vi "ManipulaEventos.vi"(10 "Error en fechas?":bool, 11 "Data In":string[][](array[string])) -> ()   [LabVIEW 2018]
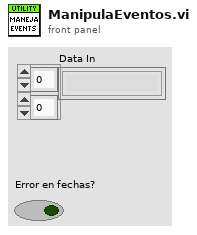
[diagram p1: front panel]
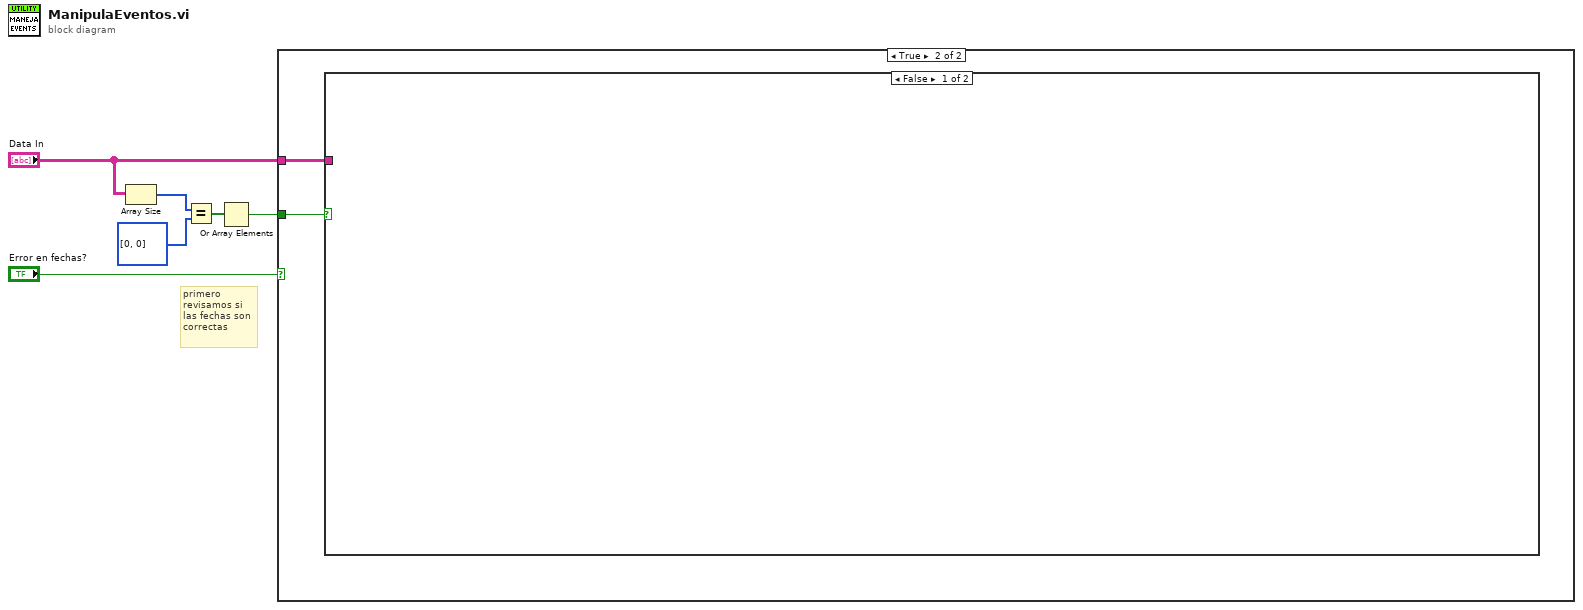
[diagram p0: block diagram]
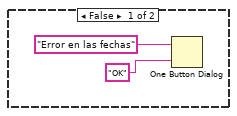
[diagram p2: hidden frame]
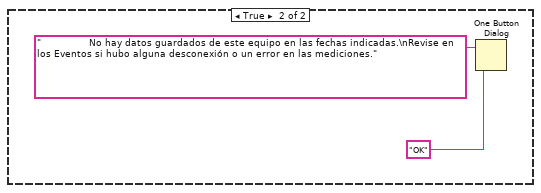
[diagram p3: hidden frame]
diagram:
  # "primero \nrevisamos si \nlas fechas son\ncorrectas"
  n1 = Array Size(array="Data In") -> (size(s)=w6:i32[])
  n2 = Equal?(x=w6, y=i32[] [0, 0] ("size(s)")) -> (x = y?=w4:bool[])
  n3 = Or Array Elements(Boolean array=w4) -> (logical OR=w3:bool)
  n4 = case shown="True" "Error en fechas?" {
    tunnel: w3 -> [_ w10]
    tunnel: "Data In" -> [_ w9]
    frame False {
      n5 = One Button Dialog(message="Error en las fechas", button name ("OK")="OK") -> ()  [unwired: 1 out]
    }
    frame True {
      n6 = case shown="False" w10 {
        tunnel: w9 -> [_ _]
        frame False {
        }
        frame True {
          n7 = One Button Dialog(message="                No hay datos guardados de este equipo en las fechas indicadas.\nRevise en los Eventos si hubo alguna desconexión o un error en las mediciones.", button name ("OK")="OK") -> ()  [unwired: 1 out]
        }
      }
    }
  }
